vi "Unlock.vi"(8 "error in":errorcluster, 11 "VISA resource name":refnum<visa-resource-name>) -> (0 "error out":errorcluster, 3 "VISA resource name out":refnum<visa-resource-name>)   [LabVIEW 2017, in "Digikrom DK24x.lvlib"]
doc: "Unlocks the VISA to terminate commands that do not return a status byte."
uses:
  Digikrom DK24x.lvlib
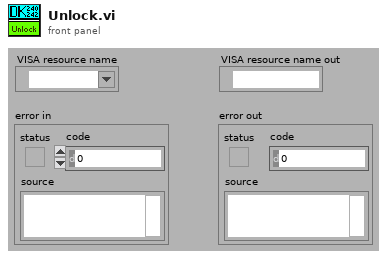
[diagram p1: front panel]
types:
  T1 = typedef "Semaphore RefNum" = refnum<k1>
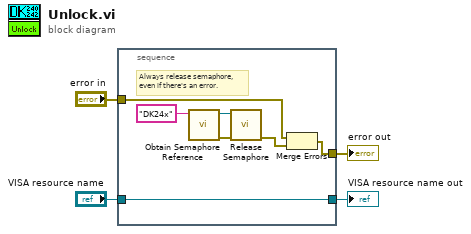
[diagram p0: block diagram]
diagram:
  n1 = stacked-sequence {
    tunnel: "error in" -> [w7]
    tunnel: [w6] -> w2
    tunnel: [w5] -> w3
    tunnel: "VISA resource name" -> [w5]
    frame #0 {
      # "Always release semaphore,\neven if there's an error."
      n2 = call <vilib>:"Obtain Semaphore Reference.vi"("name (unnamed)"="DK24x") -> ("error out"=w9:errorcluster, "semaphore"=w10:T1)  [unwired: 2 in, 3 out]
      n3 = call <vilib>:"Release Semaphore.vi"("error in (no error)"=w9, "semaphore"=w10) -> ("error out"=w8:errorcluster)  [unwired: 5 out]
      n4 = Merge Errors(w7, w8) -> (w6:errorcluster)
    }
  }
  "VISA resource name out" <- w3
  "error out" <- w2
